vi "Config ACTION.vi"(8 "error in (no error)":errorcluster, 11 "Mastering in":refnum<class "Mastering.lvclass">) -> (0 "error out":errorcluster, 3 "Mastering out":refnum<class "Mastering.lvclass">)   [LabVIEW 2014, in "SeqLoop.lvlib" / "STEP Classes.lvlib" / "Mastering.lvclass"]
uses:
  Mastering.lvclass
  Resources/XControls/Selectable ListBox xControl/ListBox XControl.xctl
  <vilib>/Utility/miscctls.llb/LVPointTypeDef.ctl
  Mastering.lvclass/Mastering.ctl
panel:
  in  "MAX(T) or MIN(F)?":bool
  in  "Deselect All":bool
  in  "Select All":bool
  in  "Cancel":bool
  in  "Save":bool
  in  "Measurement List":string[](xcontrol)
  # "Seleccione Transductores para Mastering (MAX o MIN)"
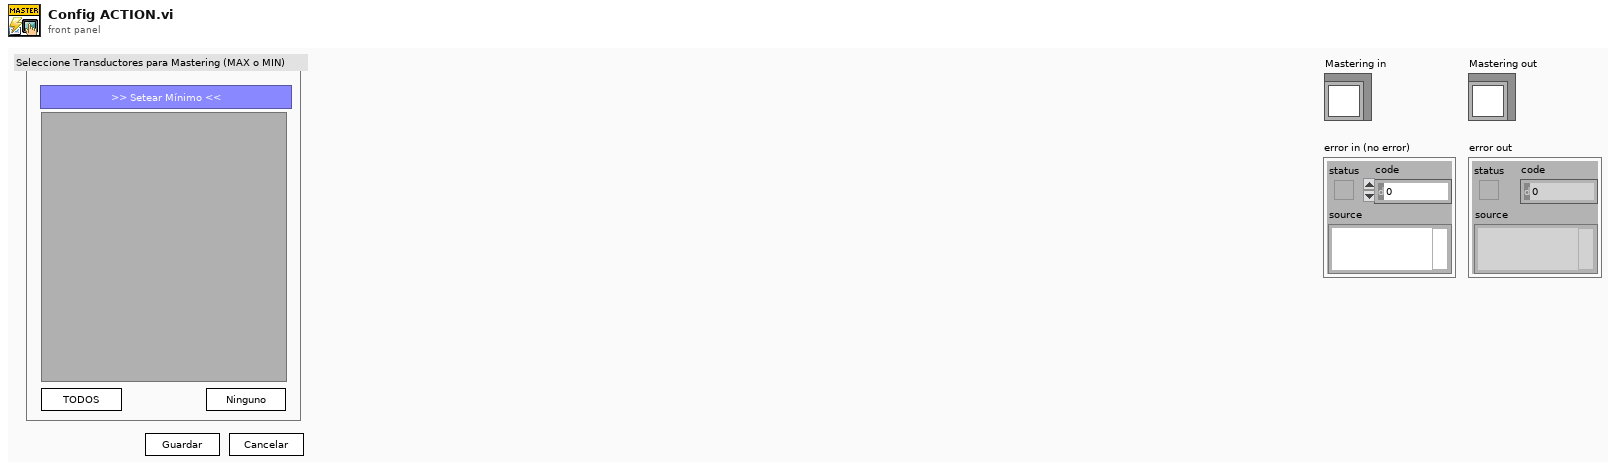
[diagram p1: front panel]
types:
  T1 = typedef "LVPointTypeDef.ctl" = cluster{"Horizontal":i16, "Vertical":i16}
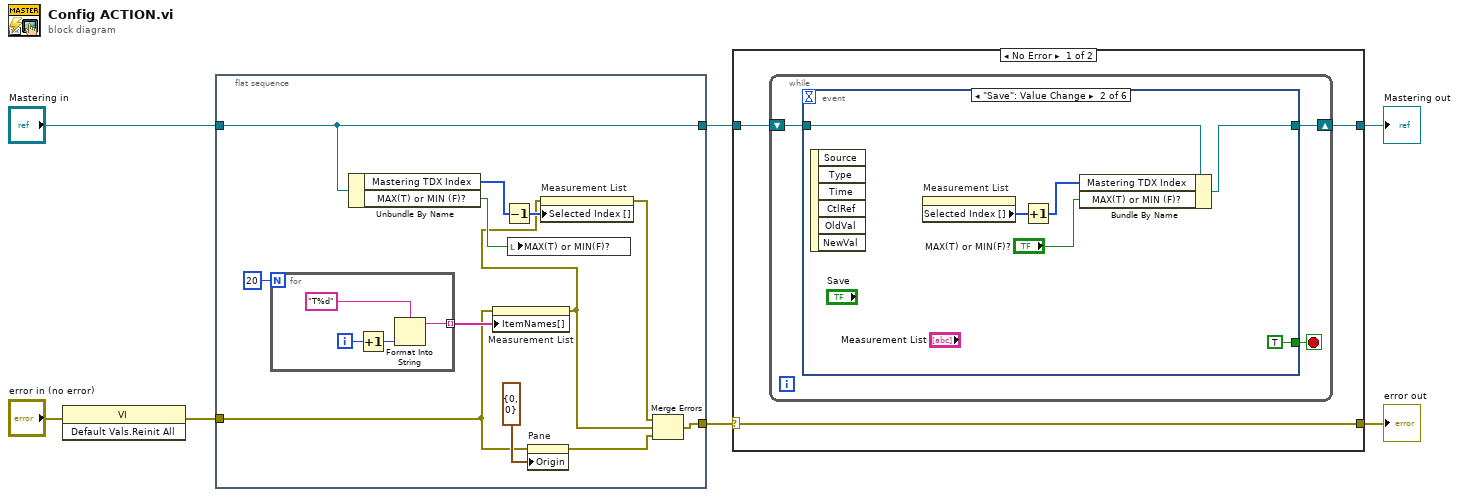
[diagram p0: block diagram]
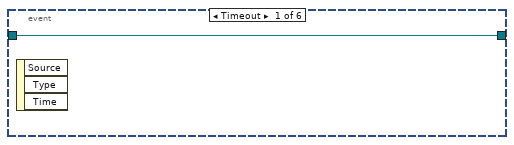
[diagram p2: hidden frame]
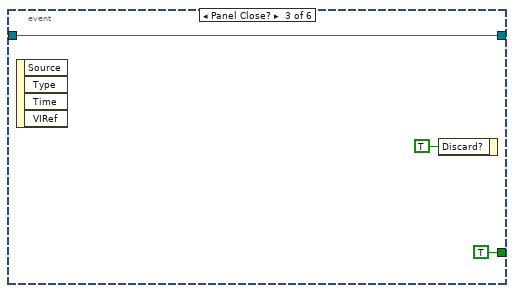
[diagram p3: hidden frame]
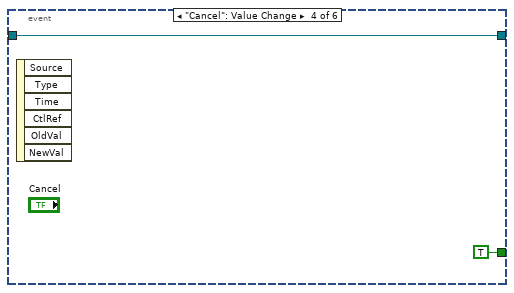
[diagram p4: hidden frame]
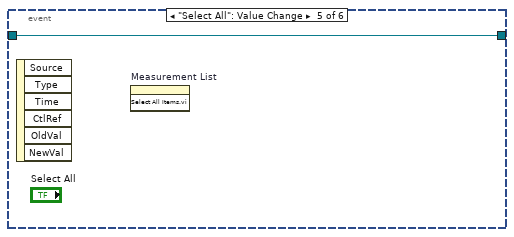
[diagram p5: hidden frame]
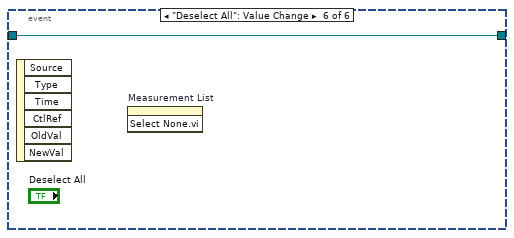
[diagram p6: hidden frame]
diagram:
  n1 = invoke class="VI" method="Default Vals.Reinit All"(error in="error in (no error)") -> (error out=w6:errorcluster)  [unwired: 2 in, 2 out]
  n2 = flat-sequence {
    tunnel: "Mastering in" -> [w13]
    tunnel: [w17] -> w7
    tunnel: w6 -> [w9]
    tunnel: [w13] -> w5
    frame #0 {
      n3 = for {
        N: 20 -> [_]
        tunnel: [w20] -> w19 mode=indexing
        i -> [w21]
        n4 = Increment(x=w21) -> (x+1=w22:i32)
        n5 = Format Into String(format string="T%d", w22) -> (resulting string=w20:string)  [unwired: 2 in, 1 out]
      }
      n6 = Unbundle By Name(w13) -> ("Mastering TDX Index"=w14:i32[], "MAX(T) or MIN (F)?"=w10:bool)
      n7 = property on="Measurement List" class="ListBox XControl (strict)"(error in=w9, "ItemNames[]"=w19) -> (error out=w8:errorcluster)  [unwired: 1 in, 1 out]
      n8 = Decrement(x=w14) -> (x-1=w15:i32[])
      n9 = local write "MAX(T) or MIN(F)?"(w10) -> ()
      n10 = property on="Pane" class="Pane"(error in=w9, "Origin"=T1 {"Horizontal"=0, "Vertical"=0}) -> (error out=w11:errorcluster)  [unwired: 1 in, 1 out]
      n11 = property on="Measurement List" class="ListBox XControl (strict)"(error in=w8, "Selected Index []"=w15) -> (error out=w16:errorcluster)  [unwired: 1 in, 1 out]
      n12 = Merge Errors(w16, w8, w11) -> (w17:errorcluster)
    }
  }
  n13 = case shown="No Error" w7 {
    selector: w7 -> [w26 w45]
    tunnel: [w26 w45] -> w1
    tunnel: [w24 w44] -> w2
    tunnel: w5 -> [w25 w44]
    frame No Error {
      n14 = while {
        shift-right: [w28] -> w24
        shift-left: w25 -> [w29]
        stop <- w27 stop-if-true
        n15 = event shown="[1] \"Save\": Value Change" {
          selector: _ -> [_ _ _ _ _ _]
          dyn-events: _ -> [_ _ _ _ _ _]
          timeout: _ -> [_ _ _ _ _ _]
          tunnel: w29 -> [w30 w35 w39 w41 w42 w43]
          tunnel: [w30 w34 w39 w41 w42 w43] -> w28
          tunnel: [_ TRUE TRUE TRUE _ _] -> w27
          event Timeout {
            n16 = event-data() -> ()  [unwired: 1 in, 3 out]
          }
          event "Save": Value Change {
            n17 = event-data() -> ()  [unwired: 1 in, 6 out]
            n18 = property on="Measurement List" class="ListBox XControl (strict)"() -> ("Selected Index []"=w33:i32[])  [unwired: 2 in, 2 out]
            n19 = Increment(x=w33) -> (x+1=w32:i32[])
            n20 = Bundle By Name(cluster=w35, "Mastering TDX Index"=w32, "MAX(T) or MIN (F)?"="MAX(T) or MIN(F)?") -> (w34:refnum<class "Mastering.lvclass">)
          }
          event Panel Close? {
            n21 = event-data() -> ()  [unwired: 1 in, 4 out]
            n22 = event-data("Discard?"=TRUE) -> ()  [unwired: 1 in, 1 out]
          }
          event "Cancel": Value Change {
            n23 = event-data() -> ()  [unwired: 1 in, 6 out]
          }
          event "Select All": Value Change {
            n24 = event-data() -> ()  [unwired: 1 in, 6 out]
            n25 = invoke on="Measurement List" class="ListBox XControl (strict)" method="Select All Items.vi"() -> ()  [unwired: 3 in, 3 out]
          }
          event "Deselect All": Value Change {
            n26 = event-data() -> ()  [unwired: 1 in, 6 out]
            n27 = invoke on="Measurement List" class="ListBox XControl (strict)" method="Select None.vi"() -> ()  [unwired: 3 in, 3 out]
          }
        }
      }
    }
    frame Error {
    }
  }
  "error out" <- w1
  "Mastering out" <- w2
